vi "Format InstanceNetworkInterfaceAttachmentType_LVXML.vi"(8 "error in (no error)":errorcluster, 10 "xmlData in":T2, 11 "AWS_EC2 in":refnum<class "AWS_EC2.lvclass">) -> (0 "error out":errorcluster, 2 "InstanceNetworkInterfaceAttachmentType":T3, 3 "AWS_EC2 out":refnum<class "AWS_EC2.lvclass">)   [LabVIEW 2014, in "AWS_EC2.lvlib" / "AWS_EC2.lvclass"]
uses:
  AWS_EC2.lvclass
  EC2 Datatypes/InstanceNetworkInterfaceAttachmentType.ctl
  lv-xml-parser/r0/trunk/VI Source/EventType.ctl
  AWS_EC2.lvlib
  lv-xml-parser/r0/trunk/VI Source/LV XML Parser.lvlib
  AWS Core Lib/VI Source/AWS_Core.lvlib
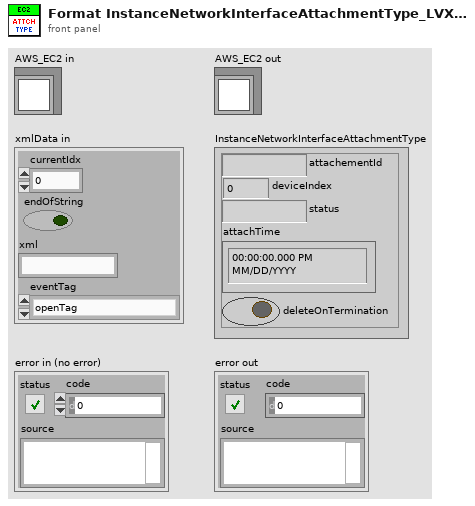
[diagram p1: front panel]
types:
  T1 = typedef "LV XML Parser.lvlib/EventType.ctl" = enum16{"openTag", "endOpenTag", "closeTag", "comment", "endComment", "endOfFile", "attribute", "startXml"}
  T2 = cluster{"currentIdx":i32, "endOfString":bool, "xml":string, "eventTag":T1}
  T3 = typedef "AWS_EC2.lvlib/InstanceNetworkInterfaceAttachmentType.ctl" = cluster{"attachementId":string, "deviceIndex":i32, "status":string, "attachTime":timestamp, "deleteOnTermination":bool}
  T4 = cluster{"namespaceUri":string, "localName":string}
  T5 = cluster{"Attributes":cluster{"localName":string, "namespaceUri":string, "value":string}[], "localName":string, "namespaceUri":string, "valueXmlData":cluster{"currentIdx":i32, "endOfString":bool, "xml":string, "eventTag":T1}}[]
  T6 = cluster{"Attributes":cluster{"localName":string, "namespaceUri":string, "value":string}[], "localName":string, "namespaceUri":string, "valueXmlData":cluster{"currentIdx":i32, "endOfString":bool, "xml":string, "eventTag":T1}}
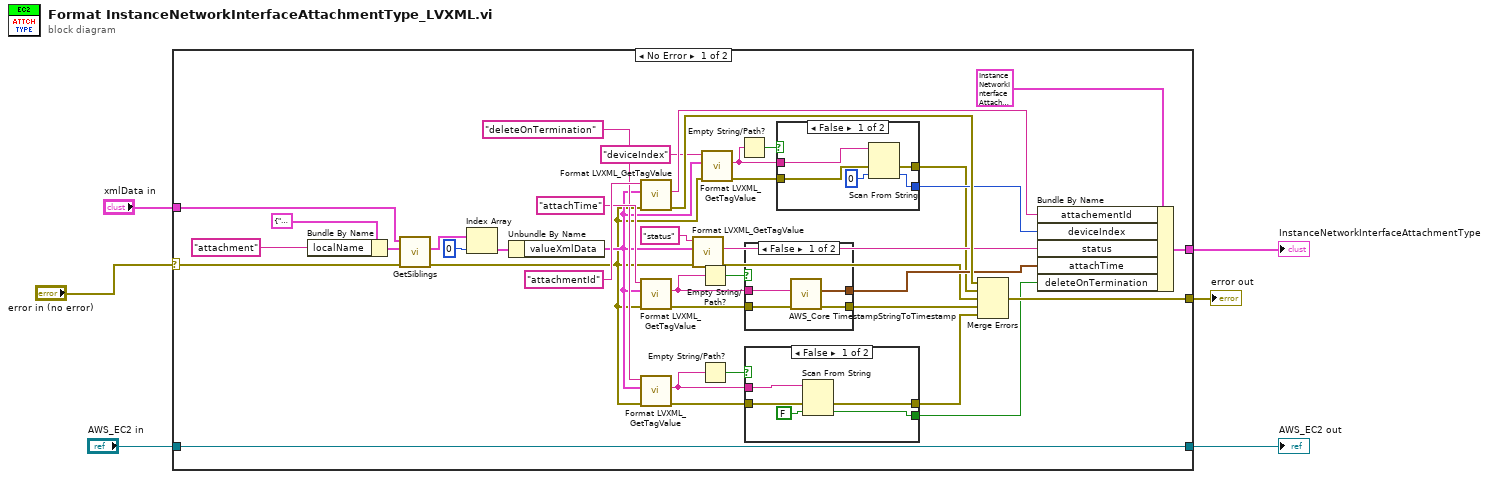
[diagram p0: block diagram]
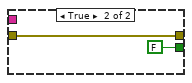
[diagram p3: hidden frame]
diagram:
  n1 = case shown="No Error" "error in (no error)" {
    selector: "error in (no error)" -> [w37 w64]
    tunnel: "xmlData in" -> [w38 _]
    tunnel: [w25 w64] -> w4
    tunnel: [w36 _] -> w6
    tunnel: [w22 w63] -> w2
    tunnel: "AWS_EC2 in" -> [w22 w63]
    frame No Error {
      n2 = Bundle By Name(cluster=T4 {"namespaceUri"="", "localName"=""} ("limitToTag"), "localName"="attachment" ("Tag name")) -> (w43:T4)
      n3 = call "GetSiblings.vi"("error in (no error)"=w37, "limitToTag"=w43, "xmlData"=w38) -> ("error out"=w15:errorcluster, "Siblings"=w40:T5)  [unwired: 7 in]
      n4 = Index Array(array=w40, index=0) -> (element=w39:T6)
      n5 = Unbundle By Name(w39) -> ("valueXmlData"=w16:T2)
      n6 = call "Format LVXML_GetTagValue.vi"("error in (no error)"=w15, "xmlDataIn"=w16, "Tag name"="attachmentId") -> ("error out"=w23:errorcluster, "Value"=w24:string)  [unwired: 6 in, 1 out]
      n7 = call "Format LVXML_GetTagValue.vi"("error in (no error)"=w15, "xmlDataIn"=w16, "Tag name"="attachTime") -> ("error out"=w26:errorcluster, "Value"=w30:string)  [unwired: 6 in, 1 out]
      n8 = call "Format LVXML_GetTagValue.vi"("error in (no error)"=w15, "xmlDataIn"=w16, "Tag name"="deleteOnTermination") -> ("error out"=w27:errorcluster, "Value"=w28:string)  [unwired: 6 in, 1 out]
      n9 = call "Format LVXML_GetTagValue.vi"("error in (no error)"=w15, "xmlDataIn"=w16, "Tag name"="status") -> ("error out"=w8:errorcluster, "Value"=w18:string)  [unwired: 6 in, 1 out]
      n10 = Empty String/Path?(string/path=w30) -> (empty?=w31:bool)
      n11 = Empty String/Path?(string/path=w28) -> (empty?=w29:bool)
      n12 = call "Format LVXML_GetTagValue.vi"("error in (no error)"=w15, "xmlDataIn"=w16, "Tag name"="deviceIndex") -> ("error out"=w13:errorcluster, "Value"=w12:string)  [unwired: 6 in, 1 out]
      n13 = Empty String/Path?(string/path=w12) -> (empty?=w14:bool)
      n14 = case shown="False" w31 {
        tunnel: w30 -> [w61 _]
        tunnel: [w60 _] -> w19
        tunnel: w26 -> [w59 w62]
        tunnel: [w58 w62] -> w9
        frame False {
          n15 = call "AWS_Core TimestampStringToTimestamp.vi"("error in"=w59, "AWS Timestamp String"=w61) -> ("error out"=w58:errorcluster, "Time Stamp Control"=w60:timestamp)  [unwired: 8 in]
        }
        frame True {
        }
      }
      n16 = case shown="False" w29 {
        tunnel: [w55 w57] -> w10
        tunnel: [w54 FALSE] -> w20
        tunnel: w27 -> [w52 w57]
        tunnel: w28 -> [w51 _]
        frame False {
          n17 = Scan From String(input string=w51, error in=w52, default 1=FALSE) -> (error out=w55:errorcluster, output 1=w54:bool)  [unwired: 2 in, 2 out]
        }
        frame True {
        }
      }
      n18 = case shown="False" w14 {
        tunnel: [w45 w50] -> w7
        tunnel: [w46 _] -> w11
        tunnel: w13 -> [w49 w50]
        tunnel: w12 -> [w48 _]
        frame False {
          n19 = Scan From String(input string=w48, error in=w49, default 1=0 ("deviceIndex")) -> (error out=w45:errorcluster, output 1=w46:i32)  [unwired: 2 in, 2 out]
        }
        frame True {
        }
      }
      n20 = Merge Errors(w23, w7, w8, w9, w10) -> (w25:errorcluster)
      n21 = Bundle By Name(cluster=T3 {"attachementId"="", "deviceIndex"=0, "status"="", "attachTime"=timestamp(0 s since 1904-01-01), "deleteOnTermination"=FALSE} ("InstanceNetworkInterfaceAttachmentType"), "attachementId"=w24, "deviceIndex"=w11, "status"=w18, "attachTime"=w19, "deleteOnTermination"=w20) -> (w36:T3)
    }
    frame Error {
    }
  }
  "InstanceNetworkInterfaceAttachmentType" <- w6
  "error out" <- w4
  "AWS_EC2 out" <- w2
